vi "FPGA-Start.vi"(3 "ServosWarmHigh (us)KaltHigh(us)":T1) -> (0 "error out":errorcluster, 1 "FPGA VI Reference Out":refnum<k20>)   [LabVIEW 2010]
uses:
  <vilib>/userDefined/High Color/nirio_resource_hc.ctl
  <vilib>/rvi/interface/nirviOpenFPGA/nirviOpenFPGA.xnode
  <vilib>/rvi/interface/nirviMethod/nirviMethod.xnode
  <vilib>/Utility/error.llb/Error Cluster From Error Code.vi
  <vilib>/LabVIEW Targets/FPGA/cRIO/shared/nicrio_ModuleControls/nicrio_cRIO-9871_FlowControlEnum.ctl
  <vilib>/LabVIEW Targets/FPGA/cRIO/shared/nicrio_ModuleControls/nicrio_cRIO-9871_StopBitsEnum.ctl
  <vilib>/LabVIEW Targets/FPGA/cRIO/shared/nicrio_ModuleControls/nicrio_cRIO-9871_ParityEnum.ctl
  <vilib>/LabVIEW Targets/FPGA/cRIO/shared/nicrio_ModuleControls/nicrio_cRIO-9871_DataBitsEnum.ctl
  <vilib>/LabVIEW Targets/FPGA/cRIO/shared/nicrio_ModuleControls/nicrio_cRIO-9871_BaudRateEnum.ctl
  <vilib>/rvi/interface/nirviReadWriteControl/nirviReadWriteControl.xnode
  C:/Users/HAGAR-IV/Desktop/Zeugs/Johnny/pertrasgc fpga/FPGA-Programm-10-14.vi
  C:/Users/HAGAR-IV/Desktop/Zeugs/markus/version feb 2012/FPGA Bitfiles/pertrasgcfpga2_FPGATarget_FPGA-Programm-10_16368CB6.lvbitx
  <vilib>/rvi/errors/niLvFpgaWhatHappensToTopLevelVI.ctl
  <vilib>/rvi/interface/common/niFpgaNodeNameForErrorReporting.ctl
  <vilib>/rvi/errors/niLvFpgaAdjustHostInterfaceError.vi
  NiFpgaLv.dll
  <vilib>/FPGAPlugInAG/cRIO-9114/niLvFpga_Reset_cRIO-9114.vi
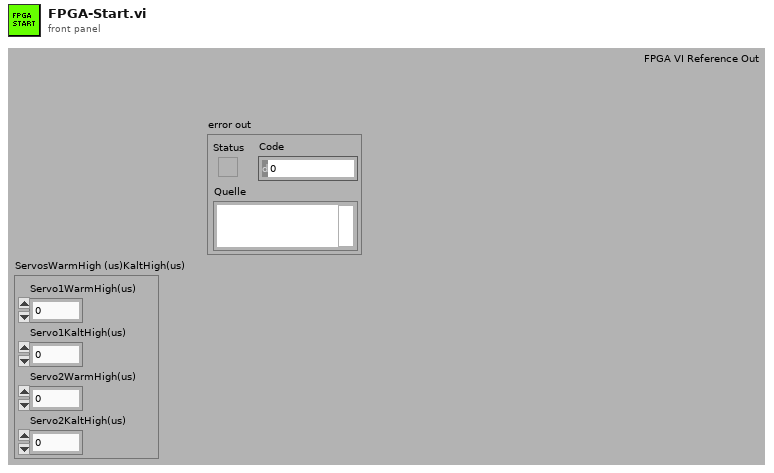
[diagram p1: front panel]
types:
  T1 = cluster{"Servo1WarmHigh(us)":u32, "Servo1KaltHigh(us)":u32, "Servo2WarmHigh(us)":u32, "Servo2KaltHigh(us)":u32}
  T2 = cluster{"MainCol1-2":u32, "Valve1-2":u32, "Spare1-2":u32, "Spare1-1":u32, "Valve1-1":u32, "MainCol1-1":u32, "Drier":u32, "Licor":u32, "ECD2":u32, "Oven2":u32, "Spare2-1":u32, "Col2-2":u32, "Col2-1":u32, "ECD1":u32}
  T3 = cluster{"MainCol1-2":bool, "Valve1-2":bool, "Spare1-2":bool, "Spare1-1":bool, "Valve1-1":bool, "MainCol1-1":bool, "Drier":bool, "Licor":bool, "ECD2":bool, "Oven2":bool, "Spare2-1":bool, "Col2-2":bool, "Col2-1":bool, "ECD1":bool}
  T4 = cluster{"Mod6/DIO 0":bool, "Mod6/DIO 1":bool, "Mod6/DIO 2":bool, "Mod6/DIO 3":bool, "Mod6/DIO 4":bool, "Mod6/DIO 5":bool, "Mod6/DIO 6":bool, "Mod6/DIO 7":bool, "Mod6/DIO 8":bool, "Mod6/DIO 9":bool, "Mod6/DIO 10":bool, "Mod6/DIO 11":bool, "Mod6/DIO 12":bool, "Mod6/DIO 13":bool, "Mod6/DIO 14":bool, "Mod6/DIO 15":bool, "Mod6/DIO 16":bool, "Mod6/DIO 17":bool, "Mod6/DIO 18":bool, "Mod6/DIO 19":bool, "Mod6/DIO 20":bool, "Mod6/DIO 21":bool, "Mod6/DIO 22":bool, "Mod6/DIO 23":bool, "Mod6/DIO 24":bool, "Mod6/DIO 25":bool, "Mod6/DIO 26":bool, "Mod6/DIO 27":bool, "Mod6/DIO 28":bool, "Mod6/DIO 29":bool, "Mod6/DIO 30":bool, "Mod6/DIO 31":bool}
  T5 = cluster{"Mod5/DIO 0":bool, "Mod5/DIO 1":bool, "Mod5/DIO 2":bool, "Mod5/DIO 3":bool, "Mod5/DIO 4":bool, "Mod5/DIO 5":bool, "Mod5/DIO 6":bool, "Mod5/DIO 7":bool, "Mod5/DIO 8":bool, "Mod5/DIO 9":bool, "Mod5/DIO 10":bool, "Mod5/DIO 11":bool, "Mod5/DIO 12":bool, "Mod5/DIO 13":bool, "Mod5/DIO 14":bool, "Mod5/DIO 15":bool, "Mod5/DIO 16":bool, "Mod5/DIO 17":bool, "Mod5/DIO 18":bool, "Mod5/DIO 19":bool, "Mod5/DIO 20":bool, "Mod5/DIO 21":bool, "Mod5/DIO 22":bool, "Mod5/DIO 23":bool, "Mod5/DIO 24":bool, "Mod5/DIO 25":bool, "Mod5/DIO 26":bool, "Mod5/DIO 27":bool, "Mod5/DIO 28":bool, "Mod5/DIO 29":bool, "Mod5/DIO 30":bool, "Mod5/DIO 31":bool}
  T6 = cluster{"proportional gain (Kc)":fxp<+/-,16,8>, "integral gain (Kc*Ts/Ti)":fxp<+/-,16,8>, "derivative gain (Kc*Td/Ts)":fxp<+/-,16,8>}
  T7 = cluster{"Per[us]Trap1":u32, "warten[us]Trap1":u32, "Per[us]Trap2":u32, "warten[us]Trap2":u32, "Per[us]Mach":u16, "vor der Messung [us]Mach":u16, "wie viele Messwerte?Mach":u16, "Abstand zwischen Messungen [us]Mach":u16}
  T8 = typedef "nicrio_cRIO-9871_BaudRateEnum.ctl" = enum16{"75 bps", "110 bps", "134 bps", "150 bps", "300 bps", "600 bps", "1200 bps", "1800 bps", "2400 bps", "4800 bps", "7200 bps", "9600 bps", "14.4 kbps", "19.2 kbps", "28.8 kbps", "38.4 kbps", "57.6 kbps", "115.2 kbps", "230.4 kbps", "460.8 kbps", "921.6 kbps"}
  T9 = typedef "nicrio_cRIO-9871_DataBitsEnum.ctl" = enum8{"5", "6", "7", "8"}
  T10 = typedef "nicrio_cRIO-9871_ParityEnum.ctl" = enum8{"None", "Odd", "Even", "Mark", "Space"}
  T11 = typedef "nicrio_cRIO-9871_StopBitsEnum.ctl" = enum8{"1", "1.5", "2"}
  T12 = typedef "nicrio_cRIO-9871_FlowControlEnum.ctl" = enum8{"None", "Software (XON / XOFF)", "Hardware (RTS / CTS)"}
  T13 = cluster{"Mod7/Port1":cluster{"Baud Rate":T8, "Data Bits":T9, "Parity":T10, "Stop Bits":T11, "Flow Control":T12}, "Mod7/Port2":cluster{"Baud Rate":T8, "Data Bits":T9, "Parity":T10, "Stop Bits":T11, "Flow Control":T12}, "Mod7/Port3":cluster{"Baud Rate":T8, "Data Bits":T9, "Parity":T10, "Stop Bits":T11, "Flow Control":T12}, "Mod7/Port4":cluster{"Baud Rate":T8, "Data Bits":T9, "Parity":T10, "Stop Bits":T11, "Flow Control":T12}, "Mod8/Port1":cluster{"Baud Rate":T8, "Data Bits":T9, "Parity":T10, "Stop Bits":T11, "Flow Control":T12}, "Mod8/Port2":cluster{"Baud Rate":T8, "Data Bits":T9, "Parity":T10, "Stop Bits":T11, "Flow Control":T12}, "Mod8/Port3":cluster{"Baud Rate":T8, "Data Bits":T9, "Parity":T10, "Stop Bits":T11, "Flow Control":T12}, "Mod8/Port4":cluster{"Baud Rate":T8, "Data Bits":T9, "Parity":T10, "Stop Bits":T11, "Flow Control":T12}}
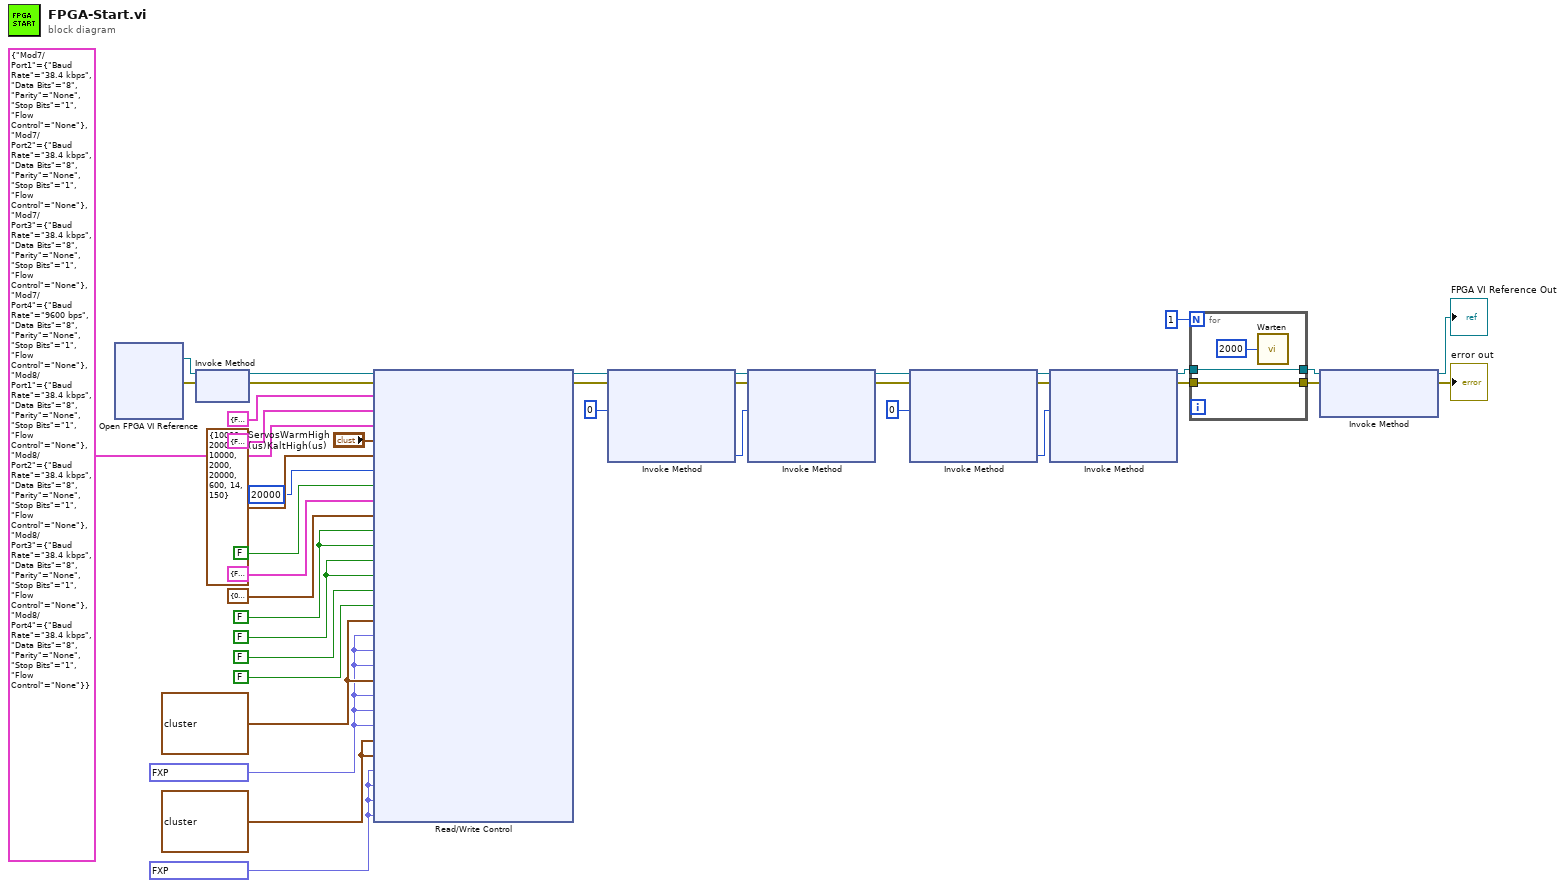
[diagram p0: block diagram]
diagram:
  w16 = fxp<+/-,16,4> 0.0 ("Umax[V]Mach1")
  w17 = T6 {"proportional gain (Kc)"=0.0, "integral gain (Kc*Ts/Ti)"=0.0, "derivative gain (Kc*Td/Ts)"=0.0} ("PIDMach1")
  w18 = fxp<+/-,16,4> 0.0 ("UTempMaxTrap1")
  w19 = T6 {"proportional gain (Kc)"=0.0, "integral gain (Kc*Ts/Ti)"=0.0, "derivative gain (Kc*Td/Ts)"=0.0} ("PIDTrap1")
  w22 = FALSE ("Heizen?Trap1")
  w23 = FALSE ("ServoTrap1kalt")
  n1 = xnode "Open FPGA VI Reference"() -> ("FPGA VI Reference Out"=w32:refnum<k20>, "error out"=w31:errorcluster)  [unwired: 2 in]
  n2 = xnode "Invoke Method"("FPGA VI Reference In"=w32, "error in"=w31) -> ("FPGA VI Reference Out"=w33:refnum<k20>, "error out"=w34:errorcluster)
  n3 = xnode "Read/Write Control"("FPGA VI Reference In"=w33, "error in"=w34, "Mod5/DIO"=T5 {"Mod5/DIO 0"=FALSE, "Mod5/DIO 1"=FALSE, "Mod5/DIO 2"=FALSE, "Mod5/DIO 3"=FALSE, "Mod5/DIO 4"=FALSE, "Mod5/DIO 5"=FALSE, "Mod5/DIO 6"=FALSE, "Mod5/DIO 7"=FALSE, "Mod5/DIO 8"=FALSE, "Mod5/DIO 9"=FALSE, "Mod5/DIO 10"=FALSE, "Mod5/DIO 11"=FALSE, "Mod5/DIO 12"=FALSE, "Mod5/DIO 13"=FALSE, "Mod5/DIO 14"=FALSE, "Mod5/DIO 15"=FALSE, "Mod5/DIO 16"=FALSE, "Mod5/DIO 17"=FALSE, "Mod5/DIO 18"=FALSE, "Mod5/DIO 19"=FALSE, "Mod5/DIO 20"=FALSE, "Mod5/DIO 21"=FALSE, "Mod5/DIO 22"=FALSE, "Mod5/DIO 23"=FALSE, "Mod5/DIO 24"=FALSE, "Mod5/DIO 25"=FALSE, "Mod5/DIO 26"=FALSE, "Mod5/DIO 27"=FALSE, "Mod5/DIO 28"=FALSE, "Mod5/DIO 29"=FALSE, "Mod5/DIO 30"=FALSE, "Mod5/DIO 31"=FALSE}, "Mod6/DIO"=T4 {"Mod6/DIO 0"=FALSE, "Mod6/DIO 1"=FALSE, "Mod6/DIO 2"=FALSE, "Mod6/DIO 3"=FALSE, "Mod6/DIO 4"=FALSE, "Mod6/DIO 5"=FALSE, "Mod6/DIO 6"=FALSE, "Mod6/DIO 7"=FALSE, "Mod6/DIO 8"=FALSE, "Mod6/DIO 9"=FALSE, "Mod6/DIO 10"=FALSE, "Mod6/DIO 11"=FALSE, "Mod6/DIO 12"=FALSE, "Mod6/DIO 13"=FALSE, "Mod6/DIO 14"=FALSE, "Mod6/DIO 15"=FALSE, "Mod6/DIO 16"=FALSE, "Mod6/DIO 17"=FALSE, "Mod6/DIO 18"=FALSE, "Mod6/DIO 19"=FALSE, "Mod6/DIO 20"=FALSE, "Mod6/DIO 21"=FALSE, "Mod6/DIO 22"=FALSE, "Mod6/DIO 23"=FALSE, "Mod6/DIO 24"=FALSE, "Mod6/DIO 25"=FALSE, "Mod6/DIO 26"=FALSE, "Mod6/DIO 27"=FALSE, "Mod6/DIO 28"=FALSE, "Mod6/DIO 29"=FALSE, "Mod6/DIO 30"=FALSE, "Mod6/DIO 31"=FALSE}, "KonfigSeriell"=T13 {"Mod7/Port1"={"Baud Rate"=enum."38.4 kbps", "Data Bits"=enum."8", "Parity"=enum."None", "Stop Bits"=enum."1", "Flow Control"=enum."None"}, "Mod7/Port2"={"Baud Rate"=enum."38.4 kbps", "Data Bits"=enum."8", "Parity"=enum."None", "Stop Bits"=enum."1", "Flow Control"=enum."None"}, "Mod7/Port3"={"Baud Rate"=enum."38.4 kbps", "Data Bits"=enum."8", "Parity"=enum."None", "Stop Bits"=enum."1", "Flow Control"=enum."None"}, "Mod7/Port4"={"Baud Rate"=enum."9600 bps", "Data Bits"=enum."8", "Parity"=enum."None", "Stop Bits"=enum."1", "Flow Control"=enum."None"}, "Mod8/Port1"={"Baud Rate"=enum."38.4 kbps", "Data Bits"=enum."8", "Parity"=enum."None", "Stop Bits"=enum."1", "Flow Control"=enum."None"}, "Mod8/Port2"={"Baud Rate"=enum."38.4 kbps", "Data Bits"=enum."8", "Parity"=enum."None", "Stop Bits"=enum."1", "Flow Control"=enum."None"}, "Mod8/Port3"={"Baud Rate"=enum."38.4 kbps", "Data Bits"=enum."8", "Parity"=enum."None", "Stop Bits"=enum."1", "Flow Control"=enum."None"}, "Mod8/Port4"={"Baud Rate"=enum."38.4 kbps", "Data Bits"=enum."8", "Parity"=enum."None", "Stop Bits"=enum."1", "Flow Control"=enum."None"}}, "ServosWarmHigh (us)KaltHigh(us)"="ServosWarmHigh (us)KaltHigh(us)", "SHFest"=T7 {"Per[us]Trap1"=10000, "warten[us]Trap1"=2000, "Per[us]Trap2"=10000, "warten[us]Trap2"=2000, "Per[us]Mach"=20000, "vor der Messung [us]Mach"=600, "wie viele Messwerte?Mach"=14, "Abstand zwischen Messungen [us]Mach"=150}, "ServosPeriode(us)"=u32 20000, "FIFO leer"=FALSE, "LHHeizen?"=T3 {"MainCol1-2"=FALSE, "Valve1-2"=FALSE, "Spare1-2"=FALSE, "Spare1-1"=FALSE, "Valve1-1"=FALSE, "MainCol1-1"=FALSE, "Drier"=FALSE, "Licor"=FALSE, "ECD2"=FALSE, "Oven2"=FALSE, "Spare2-1"=FALSE, "Col2-2"=FALSE, "Col2-1"=FALSE, "ECD1"=FALSE}, "LHPulse(us)"=T2 {"MainCol1-2"=0, "Valve1-2"=0, "Spare1-2"=0, "Spare1-1"=0, "Valve1-1"=0, "MainCol1-1"=0, "Drier"=0, "Licor"=0, "ECD2"=0, "Oven2"=0, "Spare2-1"=0, "Col2-2"=0, "Col2-1"=0, "ECD1"=0}, "ServoTrap1kalt"=w23, "ServoTrap2kalt"=w23, "Heizen?Trap1"=w22, "Heizen?Trap2"=w22, "Heizen?Mach1"=FALSE, "Heizen?Mach2"=FALSE, "PIDTrap1"=w19, "UTempMaxTrap1"=w18, "UWidrMaxTrap1"=w18, "UTempSPTrap1"=w18, "PIDTrap2"=w19, "UTempMaxTrap2"=w18, "UWidrMaxTrap2"=w18, "UTempSPTrap2"=w18, "PIDMach1"=w17, "PIDMach2"=w17, "Umax[V]Mach1"=w16, "Umax[V]Mach2"=w16, "USetp[V]Mach1"=w16, "USetp[V]Mach2"=w16) -> ("FPGA VI Reference Out"=w6:refnum<k20>, "error out"=w5:errorcluster)
  n4 = xnode "Invoke Method"("FPGA VI Reference In"=w6, "error in"=w5, "Number of Elements"=u32 0) -> ("FPGA VI Reference Out"=w38:refnum<k20>, "error out"=w35:errorcluster, "Elements Remaining"=w37:u32)  [unwired: 1 in, 1 out]
  n5 = xnode "Invoke Method"("FPGA VI Reference In"=w38, "error in"=w35, "Number of Elements"=w37) -> ("FPGA VI Reference Out"=w29:refnum<k20>, "error out"=w25:errorcluster)  [unwired: 1 in, 2 out]
  n6 = xnode "Invoke Method"("FPGA VI Reference In"=w29, "error in"=w25, "Number of Elements"=u32 0) -> ("FPGA VI Reference Out"=w27:refnum<k20>, "error out"=w24:errorcluster, "Elements Remaining"=w26:u32)  [unwired: 1 in, 1 out]
  n7 = xnode "Invoke Method"("FPGA VI Reference In"=w27, "error in"=w24, "Number of Elements"=w26) -> ("FPGA VI Reference Out"=w8:refnum<k20>, "error out"=w7:errorcluster)  [unwired: 1 in, 2 out]
  n8 = for {
    N: 1 -> [_]
    tunnel: w8 -> [w43]
    tunnel: [w43] -> w13
    tunnel: w7 -> [w42]
    tunnel: [w42] -> w11
    n9 = call "Warten"("Count(mSec)"=u32 2000) -> ()  [unwired: 1 out]
  }
  n10 = xnode "Invoke Method"("FPGA VI Reference In"=w13, "error in"=w11) -> ("FPGA VI Reference Out"=→"FPGA VI Reference Out":refnum<k20>, "error out"=→"error out":errorcluster)  [unwired: 1 in]
